vi "import variables.vi"(11 "units":string(combo)) -> (0 "Check Array":dbl[](array[numeric]), 3 "String Array From File":string[][](array[string]))   [LabVIEW 2017]
doc: "Imports from a .csv file the names and units of each variable in the order that they are collected by the program"
uses:
  <vilib>/Utility/file.llb/Read Delimited Spreadsheet (string).vi
panel:
  in  "Search String":string
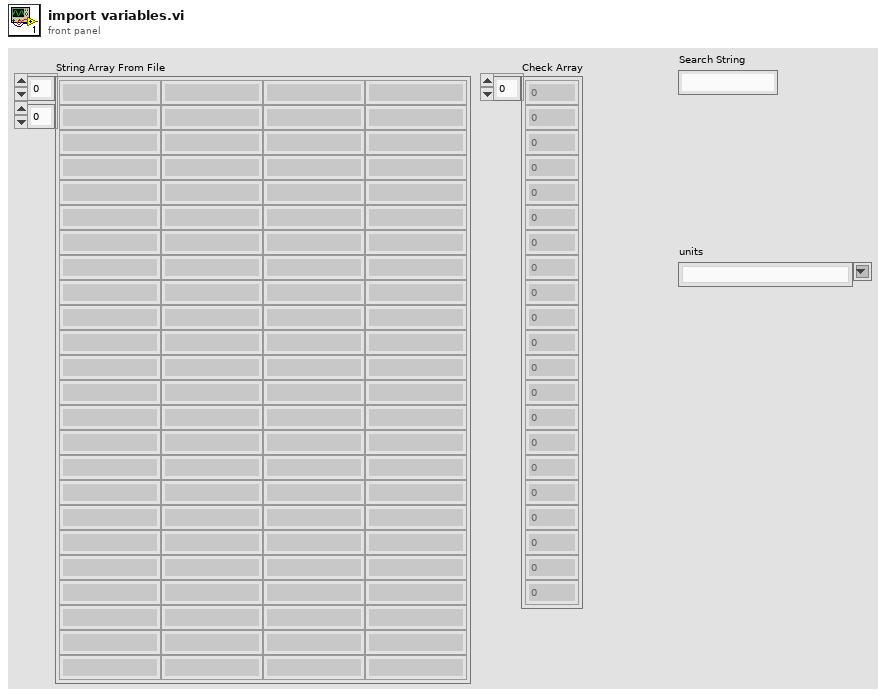
[diagram p1: front panel]
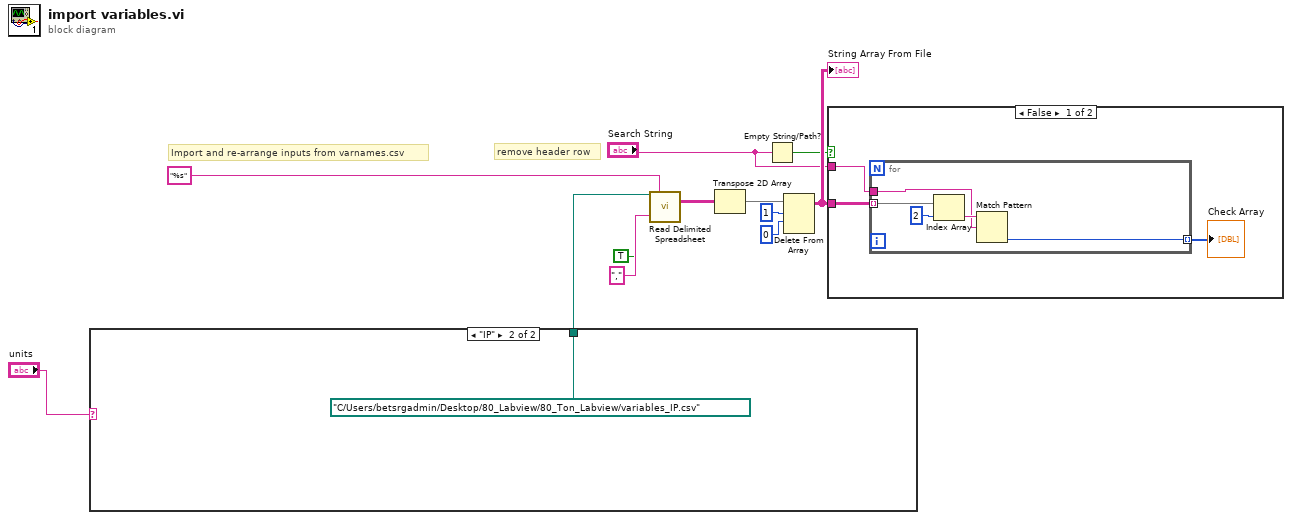
[diagram p0: block diagram]
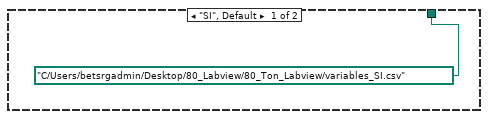
[diagram p2: hidden frame]
diagram:
  # "remove header row"
  # "Import and re-arrange inputs from varnames.csv"
  n1 = case shown="\"IP\"" "units" {
    tunnel: [path "C:/Users/betsrgadmin/Desktop/80_Labview/80_Ton_Labview/variables_SI.csv" path "C:/Users/betsrgadmin/Desktop/80_Labview/80_Ton_Labview/variables_IP.csv" ("file path (dialog if empty)")] -> w3
    frame "SI", Default {
    }
    frame "IP" {
    }
  }
  n2 = call-poly <vilib>:"Read Delimited Spreadsheet.vi"("file path (dialog if empty)"=w3, "format (%s)"="%s", "transpose? (F)"=TRUE, "delimiter (\\t)"=",") -> ("all rows"=w9:string[][])  [unwired: 6 in, 5 out]
  n3 = Transpose 2D Array(2D array=w9) -> (transposed array=w8:string[][])
  n4 = Empty String/Path?(string/path="Search String") -> (empty?=w4:bool)
  n5 = Delete From Array(array=w8, length=1, index (row)=0) -> (array with subset deleted=w5:string[][])  [unwired: 1 in, 1 out]
  "String Array From File" <- w5
  n6 = case shown="False" w4 {
    tunnel: w5 -> [w16 _]
    tunnel: "Search String" -> [w15 _]
    frame False {
      n7 = for {
        tunnel: w16 -> [w22] mode=indexing
        tunnel: [w20] -> w17 mode=indexing
        tunnel: w15 -> [w18]
        n8 = Index Array(array=w22, index=2) -> (element=w21:string)
        n9 = Match Pattern(string=w21, regular expression=w18) -> (offset past match=w20:i32)  [unwired: 1 in, 3 out]
      }
      "Check Array" <- w17
    }
    frame True {
    }
  }
